vi "PH_ImageCoG_Plotter.ProcEvents.vi"(0 "i ref in":refnum<vi>, 5 "error in":errorcluster) -> (14 "i ref out":refnum<vi>, 19 "error out":errorcluster)   [LabVIEW 2014, in "PH_ImageCoG_Plotter.lvlib"]
doc: "This method is used to define the events the object will listen to. Add your own events here."
uses:
  PH_ImageCoG_Plotter.lvlib
  CS_Core/BaseProcess/BaseProcess.event definition.ctl
  CS_Core/CAEObj/CAEObj.event definition.ctl
  CS_Core/BaseProcess/BaseProcess.descriptor string definition.ctl
  CS_Core/BaseProcess/BaseProcess.lvlib
  CS_Core/CAEObj/CAEObj.lvlib
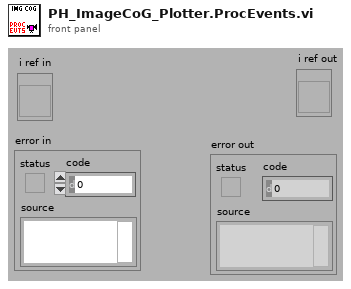
[diagram p1: front panel]
types:
  T1 = typedef "BaseProcess.lvlib/BaseProcess.event definition.ctl" = cluster{"CAEEvtDef":T2, "Data Descriptor":T3}
  T2 = typedef "CAEObj.lvlib/CAEObj.event definition.ctl" = cluster{"URL":string, "enable":bool, "ignoreResID":bool}
  T3 = typedef "BaseProcess.lvlib/BaseProcess.descriptor string definition.ctl" = string
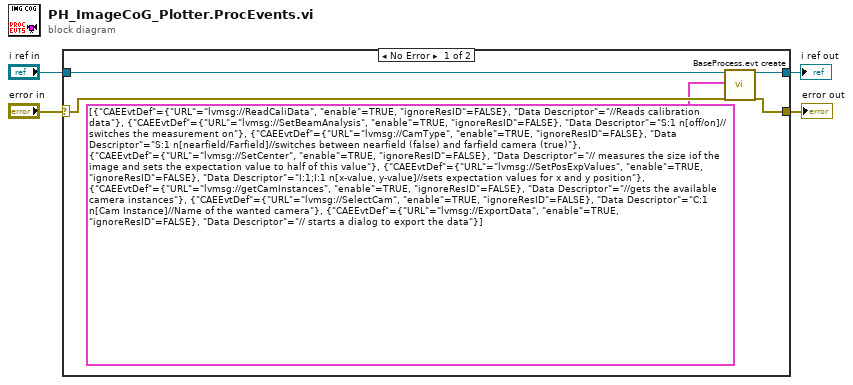
[diagram p0: block diagram]
diagram:
  n1 = case shown="No Error" "error in" {
    selector: "error in" -> [w6 w11]
    tunnel: "i ref in" -> [w9 w10]
    tunnel: [w8 w10] -> w3
    tunnel: [w7 w11] -> w2
    frame No Error {
      n2 = call "BaseProcess.evt create.vi"("i ref in"=w9, "newEvents"=T1[] [{"CAEEvtDef"={"URL"="lvmsg://ReadCaliData", "enable"=TRUE, "ignoreResID"=FALSE}, "Data Descriptor"="//Reads calibration data"}, {"CAEEvtDef"={"URL"="lvmsg://SetBeamAnalysis", "enable"=TRUE, "ignoreResID"=FALSE}, "Data Descriptor"="S:1 n[off/on]//switches the measurement on"}, {"CAEEvtDef"={"URL"="lvmsg://CamType", "enable"=TRUE, "ignoreResID"=FALSE}, "Data Descriptor"="S:1 n[nearfield/Farfield]//switches between nearfield (false) and farfield camera (true)"}, {"CAEEvtDef"={"URL"="lvmsg://SetCenter", "enable"=TRUE, "ignoreResID"=FALSE}, "Data Descriptor"="// measures the size iof the image and sets the expectation value to half of this value"}, {"CAEEvtDef"={"URL"="lvmsg://SetPosExpValues", "enable"=TRUE, "ignoreResID"=FALSE}, "Data Descriptor"="I:1;I:1 n[x-value, y-value]//sets expectation values for x and y position"}, {"CAEEvtDef"={"URL"="lvmsg://getCamInstances", "enable"=TRUE, "ignoreResID"=FALSE}, "Data Descriptor"="//gets the available camera instances"}, {"CAEEvtDef"={"URL"="lvmsg://SelectCam", "enable"=TRUE, "ignoreResID"=FALSE}, "Data Descriptor"="C:1 n[Cam Instance]//Name of the wanted camera"}, {"CAEEvtDef"={"URL"="lvmsg://ExportData", "enable"=TRUE, "ignoreResID"=FALSE}, "Data Descriptor"="// starts a dialog to export the data"}] ("new events(V3.0)"), "error in (no error)"=w6) -> ("i ref out"=w8:refnum<vi>, "error out"=w7:errorcluster)  [unwired: 13 in, 2 out]
    }
    frame Error {
    }
  }
  "i ref out" <- w3
  "error out" <- w2
